vi "FPGA Acknowledge IRQ(s).vi"   [LabVIEW 2010, in "FPGA Interface Base.lvclass"]
uses:
  <userlib>/_FPGA Interface Advanced Tools/FPGA Interface Base/FPGA Interface Base.lvclass
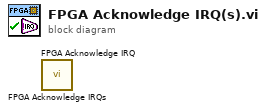
[diagram p0: block diagram]
diagram:
  n1 = call <userlib>:"FPGA Acknowledge IRQs.vi"() -> ()  [unwired: 10 in, 2 out]
  n2 = call <userlib>:"FPGA Acknowledge IRQ.vi"() -> ()  [unwired: 10 in, 2 out]
